vi "Rmv Empt Arr_2D Str.vi"(7 "조건":enum16{"행", "열", "행,열"}(ring), 8 "error in (no error)":errorcluster caption="에러 입력(에러 없음)", 11 "Data in":string[][](array[string])) -> (0 "error out":errorcluster caption="에러 출력", 3 "Data out":string[][](array[string]))   [LabVIEW 2020]
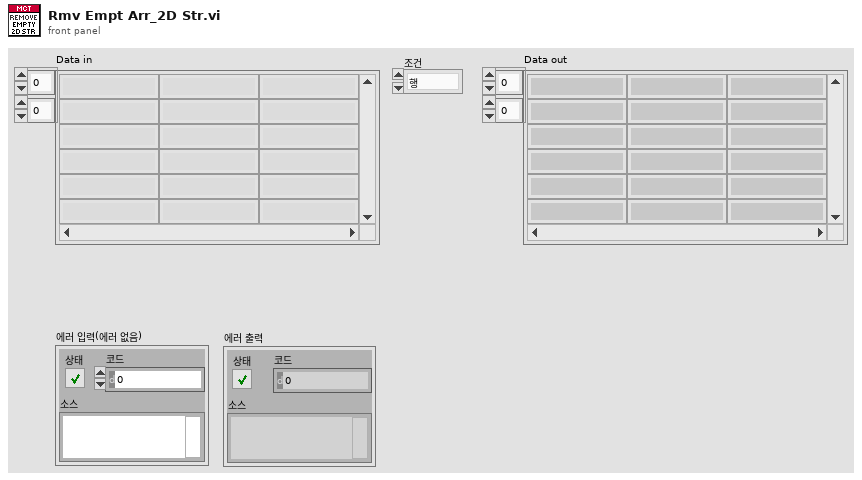
[diagram p1: front panel]
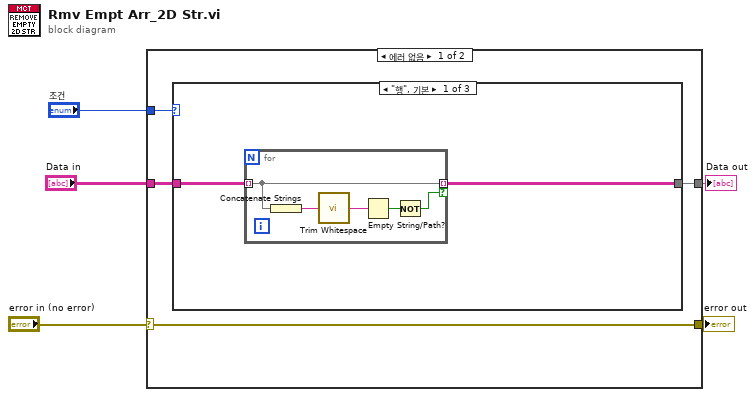
[diagram p0: block diagram]
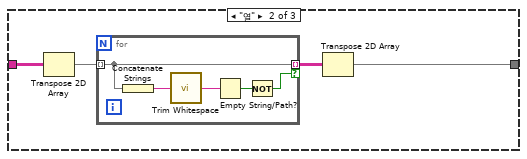
[diagram p2: hidden frame]
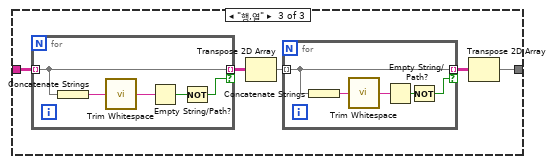
[diagram p3: hidden frame]
diagram:
  n1 = case shown="에러 없음" "error in (no error)" {
    selector: "error in (no error)" -> [w6 w42]
    tunnel: "Data in" -> [w9 w41]
    tunnel: [w8 w41] -> w4
    tunnel: "조건" -> [w7 _]
    tunnel: [w6 w42] -> w1
    frame No Error {
      n2 = case shown="\"행\", 기본" w7 {
        tunnel: w9 -> [w11 w20 w30]
        tunnel: [w10 w17 w26] -> w8
        frame "행", Default {
          n3 = for {
            tunnel: w11 -> [w14] mode=indexing
            tunnel: [w14] -> w10 mode=indexing if=w12
            n4 = Concatenate Strings(w14) -> (w16:string)
            n5 = call <vilib>:"Trim Whitespace.vi"("string"=w16) -> ("trimmed string"=w15:string)  [unwired: 1 in]
            n6 = Empty String/Path?(string/path=w15) -> (empty?=w13:bool)
            n7 = Not(x=w13) -> (.not. x?=w12:bool)
          }
        }
        frame "열" {
          n8 = Transpose 2D Array(2D array=w20) -> (transposed array=w18:string[][])
          n9 = for {
            tunnel: w18 -> [w23] mode=indexing
            tunnel: [w23] -> w19 mode=indexing if=w21
            n10 = Concatenate Strings(w23) -> (w25:string)
            n11 = call <vilib>:"Trim Whitespace.vi"("string"=w25) -> ("trimmed string"=w24:string)  [unwired: 1 in]
            n12 = Empty String/Path?(string/path=w24) -> (empty?=w22:bool)
            n13 = Not(x=w22) -> (.not. x?=w21:bool)
          }
          n14 = Transpose 2D Array(2D array=w19) -> (transposed array=w17:string[][])
        }
        frame "행,열" {
          n15 = for {
            tunnel: w30 -> [w38] mode=indexing
            tunnel: [w38] -> w27 mode=indexing if=w36
            n16 = Concatenate Strings(w38) -> (w40:string)
            n17 = call <vilib>:"Trim Whitespace.vi"("string"=w40) -> ("trimmed string"=w39:string)  [unwired: 1 in]
            n18 = Empty String/Path?(string/path=w39) -> (empty?=w37:bool)
            n19 = Not(x=w37) -> (.not. x?=w36:bool)
          }
          n20 = Transpose 2D Array(2D array=w27) -> (transposed array=w28:string[][])
          n21 = for {
            tunnel: w28 -> [w33] mode=indexing
            tunnel: [w33] -> w29 mode=indexing if=w31
            n22 = Concatenate Strings(w33) -> (w35:string)
            n23 = call <vilib>:"Trim Whitespace.vi"("string"=w35) -> ("trimmed string"=w34:string)  [unwired: 1 in]
            n24 = Empty String/Path?(string/path=w34) -> (empty?=w32:bool)
            n25 = Not(x=w32) -> (.not. x?=w31:bool)
          }
          n26 = Transpose 2D Array(2D array=w29) -> (transposed array=w26:string[][])
        }
      }
    }
    frame Error {
    }
  }
  "Data out" <- w4
  "error out" <- w1
